vi "ExSubCenterFlag.vi"(0 "Binning \nUser = 1\nCenter = 2\nFull = 3":u32=1 min=1 max=3 step=1) -> ()   [LabVIEW 2010]
uses:
  GlobalBin2x.vi
  GlobalFullBin.vi
  GlobalUserBin.vi
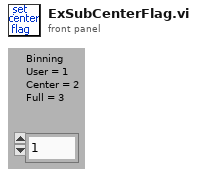
[diagram p1: front panel]
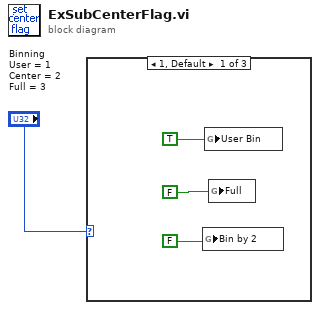
[diagram p0: block diagram]
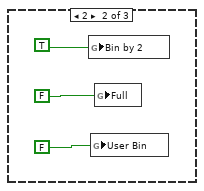
[diagram p2: hidden frame]
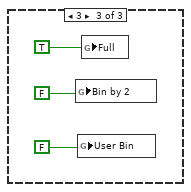
[diagram p3: hidden frame]
diagram:
  n1 = case shown="1, Default" "Binning \nUser = 1\nCenter = 2\nFull = 3" {
    frame 1, Default {
      n2 = global write "GlobalBin2x.vi" "Bin by 2"(FALSE) -> ()
      n3 = global write "GlobalUserBin.vi" "User Bin"(TRUE) -> ()
      n4 = global write "GlobalFullBin.vi" "Full"(FALSE) -> ()
    }
    frame 2 {
      n5 = global write "GlobalBin2x.vi" "Bin by 2"(TRUE) -> ()
      n6 = global write "GlobalUserBin.vi" "User Bin"(FALSE) -> ()
      n7 = global write "GlobalFullBin.vi" "Full"(FALSE) -> ()
    }
    frame 3 {
      n8 = global write "GlobalBin2x.vi" "Bin by 2"(FALSE) -> ()
      n9 = global write "GlobalUserBin.vi" "User Bin"(FALSE) -> ()
      n10 = global write "GlobalFullBin.vi" "Full"(TRUE) -> ()
    }
  }
